vi "RnachT.vi"(1 "R":dbl=11430.0 format="%.2f", 2 "Sensor Cal #":u16(ring) items=["leer", "LS 27120", "R4", "R6", "MK1-RuOx Oxfd", "Allan Bradley MK 2"]) -> (0 "T (K)":dbl=0.00957168277075326 format="%^.3e")   [LabVIEW 2010]
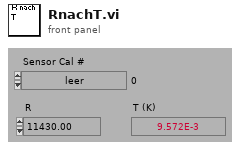
[diagram p1: front panel]
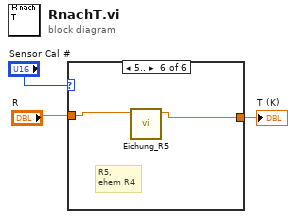
[diagram p0: block diagram]
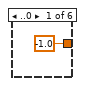
[diagram p2: hidden frame]
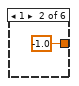
[diagram p3: hidden frame]
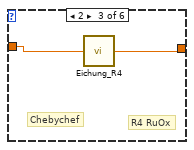
[diagram p4: hidden frame]
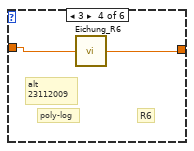
[diagram p5: hidden frame]
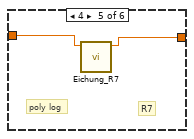
[diagram p6: hidden frame]
diagram:
  n1 = case shown="5.." "Sensor Cal #" {
    tunnel: "R" -> [_ _ w7 w9 w11 w12]
    tunnel: [-1.0 ("T (K)") -1.0 ("T (K)") w6 w8 w10 w13] -> w2
    frame ..0 {
    }
    frame 1 {
    }
    frame 2 {
      # "R4 RuOx"
      # "Chebychef"
      n2 = call "Eichung_R4.vi"("R (Ohm)"=w7) -> ("T (K)"=w6:dbl)
    }
    frame 3 {
      # "alt\n23112009"
      # "R6"
      # "poly-log"
      n3 = call "Eichung_R6.vi"("R (Ohm)"=w9) -> ("T (K)"=w8:dbl)
    }
    frame 4 {
      # "R7"
      # "poly log"
      n4 = call "Eichung_R7.vi"("R (Ohm)"=w11) -> ("T (K)"=w10:dbl)  [unwired: 10 in]
    }
    frame 5.. {
      # "R5,\nehem R4"
      n5 = call "Eichung_R5.vi"("R (Ohm)"=w12) -> ("T (K)"=w13:dbl)  [unwired: 10 in]
    }
  }
  "T (K)" <- w2
